vi "Untitled 1.vi"() -> ()   [LabVIEW 2017]
uses:
  <vilib>/Instr/_visa.llb/Select Event Type.ctl
  <vilib>/Instr/_visa.llb/VISA Configure Serial Port (Instr).vi
  <vilib>/Utility/file.llb/Write Delimited Spreadsheet (string).vi
panel:
  in  "baud rate (9600)":u32=1200
  out "波形图表":sgl[](graph)
  out "读取缓冲区":string
  in  "导入文本":bool
  in  "导入表格":bool
  in  "文本路径":path
  in  "清空接收":bool
  in  "表格路径":path
  out "x+y":u32
  in  "stop 3":bool
  out "read buffer":string
  in  "data bits (8)":u16=8 min=5 max=8 step=1
  in  "parity (0:none)":enum16{"None", "Odd", "Even", "Mark", "Space"}(ring)
  in  "stop bits (10: 1 bit)":u16(ring)=10 items=["1.0"=10, "1.5"=15, "2.0"=20]
  in  "write buffer":string
  in  "OK Button":bool
  in  "VISA resource name":refnum<visa-resource-name>
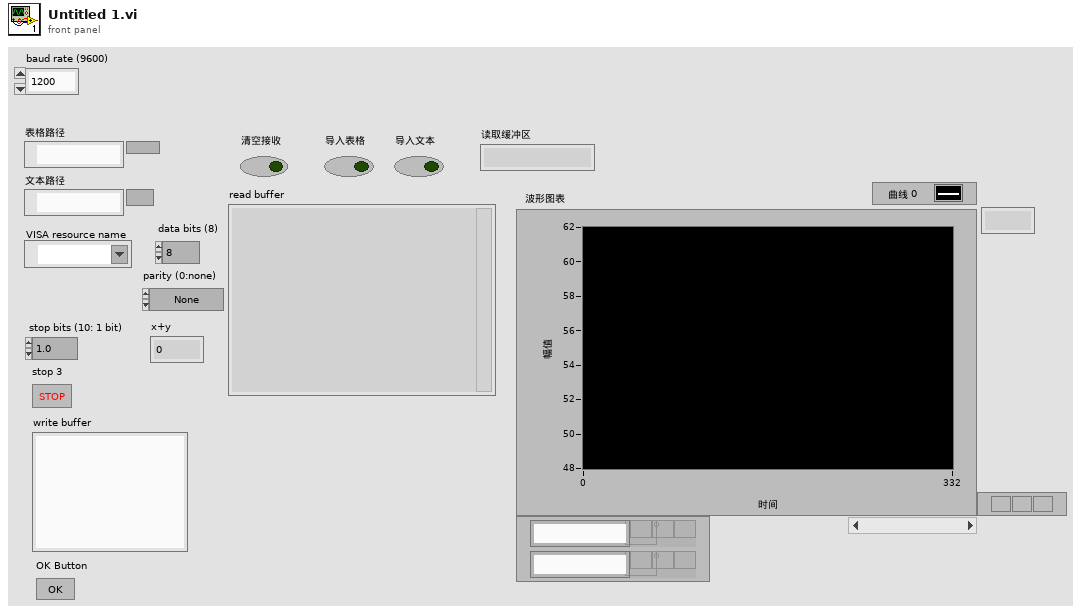
[diagram p1: front panel]
types:
  T1 = typedef "Select Event Type.ctl" = u32
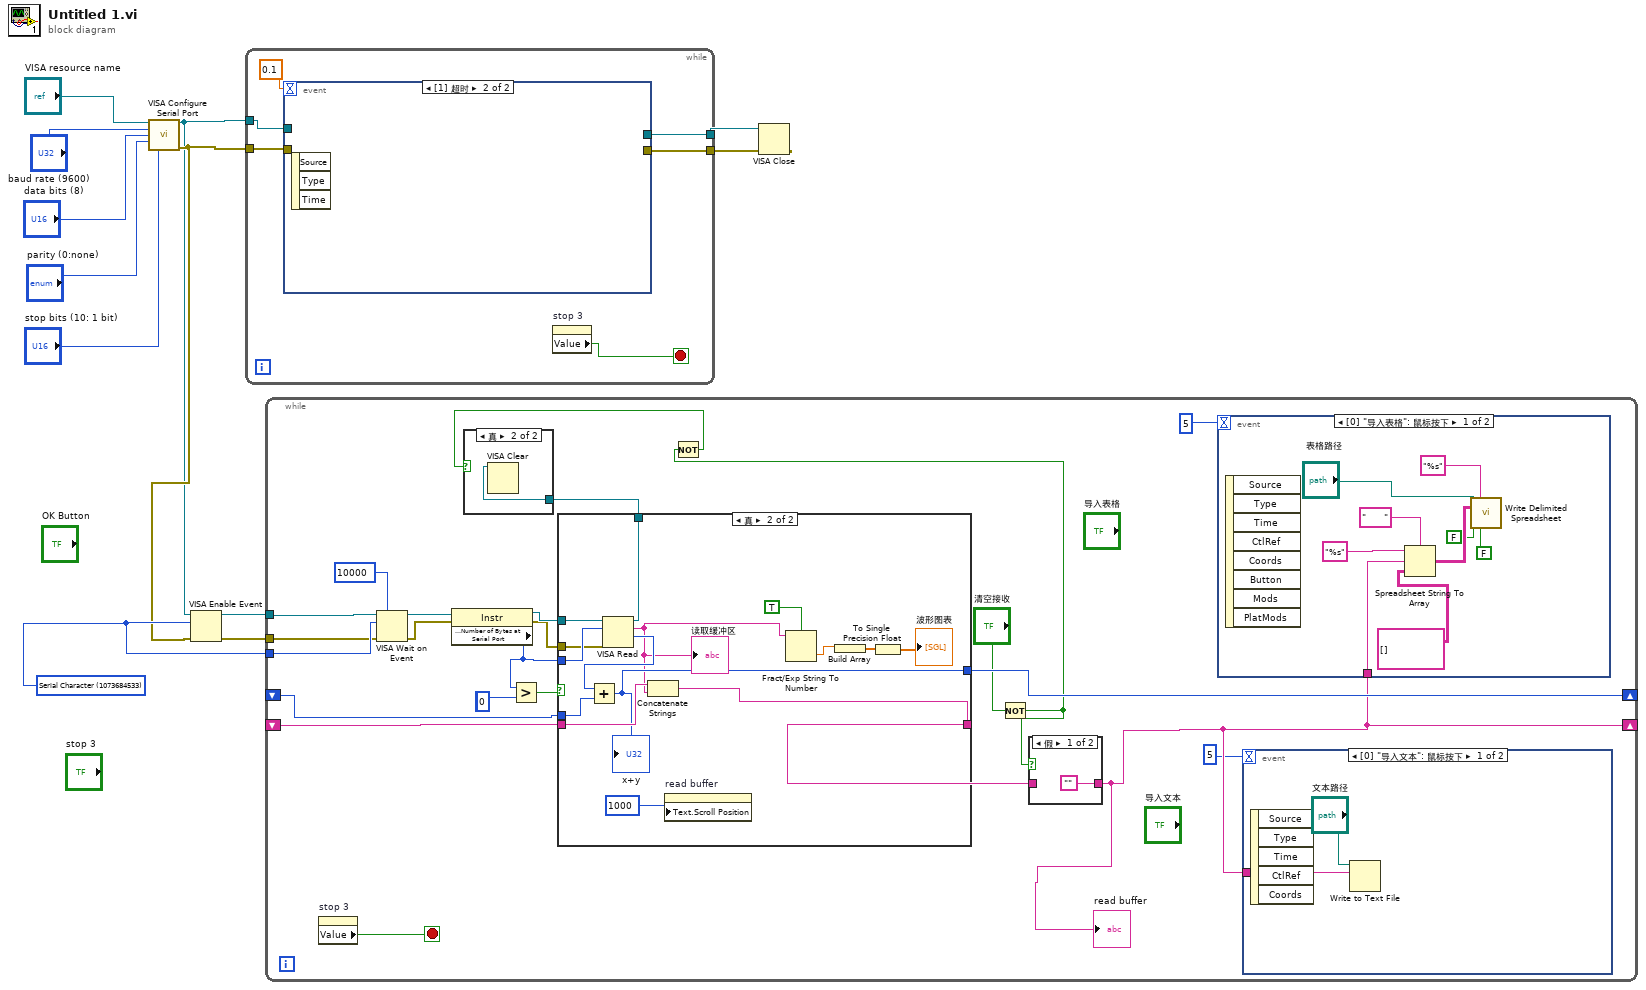
[diagram p0: block diagram]
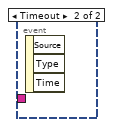
[diagram p2: hidden frame]
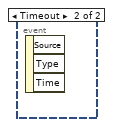
[diagram p5: hidden frame]
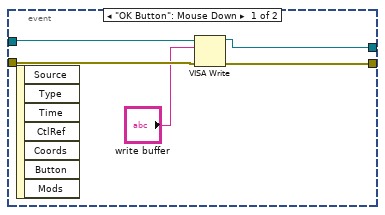
[diagram p7: hidden frame]
diagram:
  w4 = T1 1073684533 items=["Service Request"=1073684491, "Trigger"=3221168138, "Clear"=1073684493, "VXI Signal"=1073684512, "VXI/VME Interrupt"=3221168161, "VXI/VME Sysfail"=1073684509, "VXI/VME Sysreset"=1073684510, "GPIB CIC"=1073684498, "GPIB Talk"=1073684499, "GPIB Listen"=1073684500, "PXI Interrupt"=1073684514, "Serial Break"=1073684515, "Serial TermChar"=1073684516, "Serial CTS"=1073684521, "Serial DSR"=1073684522, "Serial DCD"=1073684524, "Serial RI"=1073684526, "Serial Character"=1073684533, "USB Interrupt"=1073684535, "All Enabled"=1073709055] ("Event Type")
  n1 = call-poly "VISA Configure Serial Port"("VISA resource name"="VISA resource name", "baud rate (9600)"="baud rate (9600)", "data bits (8)"="data bits (8)", "parity (0:none)"="parity (0:none)", "stop bits (10: 1 bit)"="stop bits (10: 1 bit)") -> ("VISA resource name out"=w1:refnum<visa-resource-name>, "error out"=w2:errorcluster)  [unwired: 9 in]
  n2 = VISA Enable Event(8:w2, 10:w4, 11:w1) -> (0:w3:errorcluster, 3:w5:refnum<visa-resource-name>)  [unwired: 1 in]
  n3 = while {
    tunnel: w2 -> [w18]
    tunnel: w1 -> [w17]
    tunnel: [w16] -> w11
    tunnel: [w15] -> w10
    stop <- w13 stop-if-true
    n4 = event shown="[1] 超时" {
      selector: _ -> [_ _]
      dyn-events: _ -> [_ _]
      timeout: 0.1 -> [_ _]
      tunnel: w18 -> [w23 _]
      tunnel: w17 -> [w22 _]
      tunnel: [w21 _] -> w16
      tunnel: [w20 _] -> w15
      event "OK Button": Mouse Down {
        n5 = event-data() -> ()  [unwired: 1 in, 7 out]
        n6 = VISA Write(VISA resource name=w22, write buffer="write buffer", error in (no error)=w23) -> (VISA resource name out=w21:refnum<visa-resource-name>, error out=w20:errorcluster)  [unwired: 1 out]
      }
      event Timeout {
        n7 = event-data() -> ()  [unwired: 1 in, 3 out]
      }
    }
    n8 = property on="stop 3" class="Bool (严格)"() -> ("Value"=w13:bool)  [unwired: 2 in, 2 out]
  }
  n9 = while {
    tunnel: w5 -> [w46]
    tunnel: w4 -> [w45]
    tunnel: w3 -> [w44]
    shift-right: [w25] -> _
    shift-left: _ -> [w42]
    shift-right: [w40] -> _
    shift-left: _ -> [w41]
    stop <- w43 stop-if-true
    (unwired) 0
    n10 = property on="stop 3" class="Bool (严格)"() -> ("Value"=w43:bool)  [unwired: 2 in, 2 out]
    n11 = VISA Wait on Event(7:10000, 8:w44, 10:w45, 11:w46) -> (0:w38:errorcluster, 3:w39:refnum<visa-resource-name>)  [unwired: 1 in, 2 out]
    n12 = property class="Instr"(reference=w39, error in=w38) -> (reference out=w37:refnum<visa-resource-name>, error out=w36:errorcluster, "Serial Settings:Number of Bytes at Serial Port"=w34:u32)
    n13 = Greater?(x=w34, y=0) -> (0:w35:bool)
    n14 = case shown="真" w35 {
      tunnel: w37 -> [w61 w70]
      tunnel: w34 -> [w62 w78]
      tunnel: w36 -> [_ w77]
      tunnel: w42 -> [w63 w75]
      tunnel: [w63 w71] -> w30
      tunnel: w41 -> [_ w74]
      tunnel: [w62 w73] -> w40
      tunnel: [w61 w69] -> w29
      frame False {
      }
      frame True {
        n15 = VISA Read(VISA resource name=w70, byte count=w78, error in (no error)=w77) -> (VISA resource name out=w69:refnum<visa-resource-name>, read buffer=w67:string, return count=w76:u32)  [unwired: 1 out]
        "读取缓冲区" <- w67
        n16 = Add(x=w76, y=w74) -> (x+y=w73:u32)
        "x+y" <- w73
        n17 = Concatenate Strings(w75, w67) -> (w71:string)
        n18 = property on="read buffer" class="Str"("Text.Scroll Position"=1000) -> ()  [unwired: 2 in, 2 out]
        n19 = Fract/Exp String To Number(use system decimal point (T)=TRUE ("使用系统小数点(T)"), string=w67) -> (number=w65:dbl)  [unwired: 2 in, 1 out]
        n20 = Build Array(w65) -> (w68:dbl[])
        n21 = To Single Precision Float(number=w68) -> (single precision float=→"波形图表":sgl[])
      }
    }
    n22 = Not(x="清空接收") -> (.not. x?=w27:bool)
    n23 = Not(x=w27) -> (.not. x?=w28:bool)
    n24 = case shown="真" w28 {
      tunnel: w29 -> [_ w49]
      frame False {
      }
      frame True {
        n25 = VISA Clear(VISA resource name=w49) -> ()  [unwired: 1 in, 2 out]
      }
    }
    n26 = case shown="假" w27 {
      tunnel: w30 -> [_ w51]
      tunnel: ["" w51] -> w25
      frame False {
      }
      frame True {
      }
    }
    "read buffer" <- w25
    n27 = event shown="[0] \"导入表格\": 鼠标按下" {
      selector: _ -> [_ _]
      dyn-events: _ -> [_ _]
      timeout: 5 -> [_ _]
      tunnel: w25 -> [w56 _]
      event "导入表格": Mouse Down {
        n28 = event-data() -> ()  [unwired: 1 in, 8 out]
        n29 = Spreadsheet String To Array(delimiter (Tab)="      ", format string="%s", spreadsheet string=w56, array type (2D Dbl)=string[][] []) -> (array=w54:string[][])
        n30 = call-poly <vilib>:"Write Delimited Spreadsheet.vi"("file path (dialog if empty)"="表格路径", "format (%s)"="%s" ("format (%.3f)"), "2D data"=w54, "append to file? (new file:F)"=FALSE, "transpose? (no:F)"=FALSE) -> ()  [unwired: 9 in, 2 out]
      }
      event Timeout {
        n31 = event-data() -> ()  [unwired: 1 in, 3 out]
      }
    }
    n32 = event shown="[0] \"导入文本\": 鼠标按下" {
      selector: _ -> [_ _]
      dyn-events: _ -> [_ _]
      timeout: 5 -> [_ _]
      tunnel: w25 -> [w47 _]
      event "导入文本": Mouse Down {
        n33 = event-data() -> ()  [unwired: 1 in, 5 out]
        n34 = Write to Text File(file (use dialog)="文本路径", text=w47) -> ()  [unwired: 2 in, 3 out]
      }
      event Timeout {
        n35 = event-data() -> ()  [unwired: 1 in, 3 out]
      }
    }
  }
  n36 = VISA Close(VISA resource name=w11, error in (no error)=w10) -> ()  [unwired: 1 out]
